vi "ODE_omega.vi"() -> ()   [LabVIEW 2018]
uses:
  <vilib>/imath/engines/lvmath2/RunTimeEngine/BuiltInFunctions/inv/NIMS_inv(GM).vi
  <instcachedir>/0/NIMS_inv(GM)_A6DF8FE880224208AACFE4CF9F659502.lvgen/NIMS_inv(GM)_A6DF8FE880224208AACFE4CF9F659502_000.vi
  <vilib>/imath/engines/lvmath2/RunTimeEngine/ErrorHandling/NIMS_Error From Error Code.vi
  <vilib>/imath/engines/lvmath2/RunTimeEngine/IndexRead/NIMS V(S).vi
  <instcachedir>/0/NIMS V(S)_0488751826AF41519A22953C041130DC.lvgen/NIMS V(S)_0488751826AF41519A22953C041130DC_002.vi
  <vilib>/imathl/engines/lvmath/Functions/Error Handling/Create Error.vi
  <vilib>/imath/engines/lvmath2/RunTimeEngine/ErrorHandling/NIMS_Create Error From Enums.vi
  <vilib>/imath/engines/lvmath2/RunTimeEngine/ArithmeticOperatorToken/NIMS_ArithmeticOperator_multmx-internal.vi
  <instcachedir>/0/NIMS_ArithmeticOperator_multmx-internal_16A6E1DA326644AB974D30232E729C42.lvgen/NIMS_ArithmeticOperator_multmx-internal_16A6E1DA326644AB974D30232E729C42_008.vi
  <vilib>/imath/engines/lvmath2/RunTimeEngine/ArithmeticOperatorToken/NIMS_ArithmeticOperator_multmx(M,CV)-internal.vi
  <instcachedir>/0/NIMS_ArithmeticOperator_multmx(M,CV)-internal_5287250D8D1D4A3E9F77F5DF08D432E0.lvgen/NIMS_ArithmeticOperator_multmx(M,CV)-internal_5287250D8D1D4A3E9F77F5DF08D432E0_003.vi
  <instcachedir>/0/NIMS_ArithmeticOperator_multmx(M,CV)-internal_5287250D8D1D4A3E9F77F5DF08D432E0.lvgen/NIMS_ArithmeticOperator_multmx(M,CV)-internal_5287250D8D1D4A3E9F77F5DF08D432E0_000.vi
  <vilib>/imath/engines/lvmath2/RunTimeEngine/ArithmeticOperatorToken/NIMS_ArithmeticOperator_multmx(M,CV).vi
  <instcachedir>/0/NIMS_ArithmeticOperator_multmx(M,CV)_2F1CD6A2FE4F4213A4AD1C901C2750F5.lvgen/NIMS_ArithmeticOperator_multmx(M,CV)_2F1CD6A2FE4F4213A4AD1C901C2750F5_000.vi
  <vilib>/imath/engines/lvmath2/RunTimeEngine/IndexRead/NIMS M(S).vi
  <instcachedir>/0/NIMS M(S)_B826C018497E4940AE96BD27B540B6FB.lvgen/NIMS M(S)_B826C018497E4940AE96BD27B540B6FB_000.vi
  <vilib>/imath/engines/lvmath2/RunTimeEngine/NodeEndStatement/NIMS_NodeEndStatement_Output.vi
  <instcachedir>/0/NIMS_NodeEndStatement_Output_53EC0D466D134D7ABD903AC30B43404B.lvgen/NIMS_NodeEndStatement_Output_53EC0D466D134D7ABD903AC30B43404B_005.vi
  <vilib>/imath/engines/lvmath2/RunTimeEngine/ErrorHandling/NIMS_Finalize Error.vi
  <vilib>/gmath/NI_Gmath.lvlib
panel:
  out "appended array":dbl[](array[numeric])
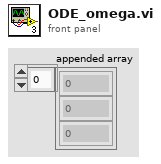
[diagram p1: front panel]
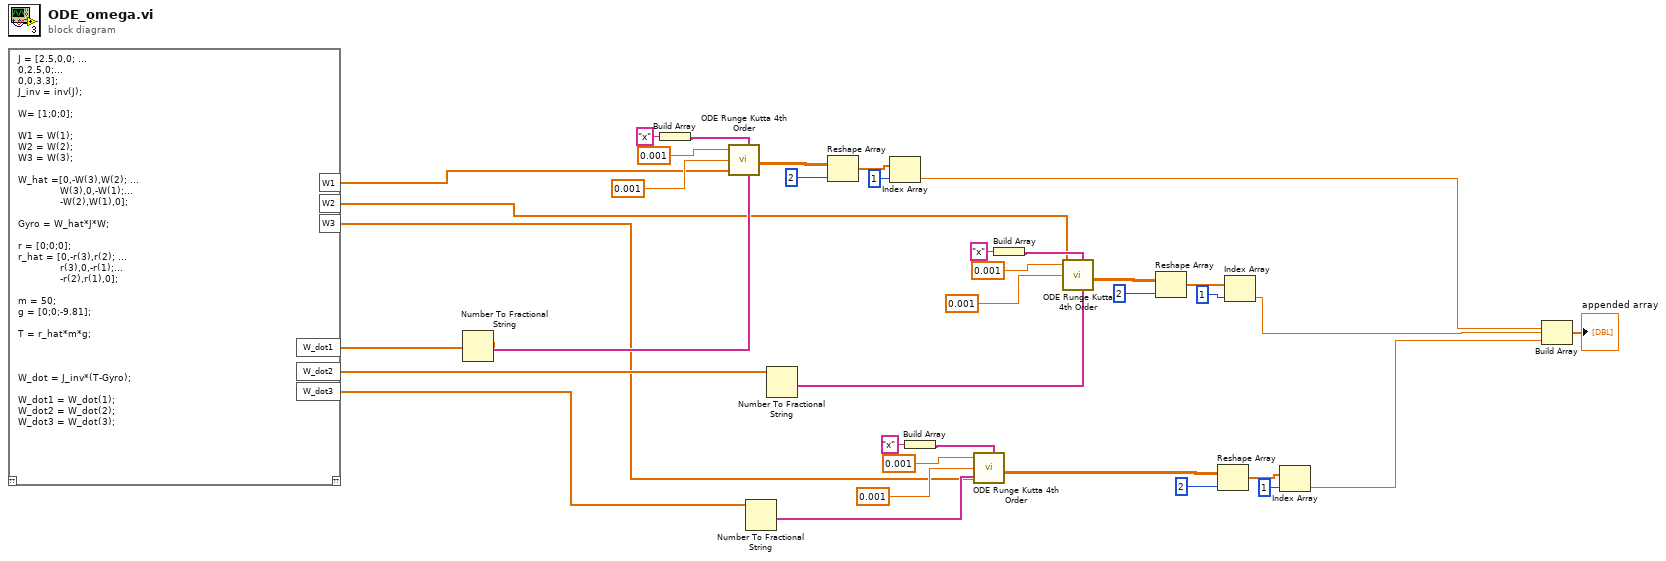
[diagram p0: block diagram]
diagram:
  n1 = mathscript code="J = [2.5,0,0; ...\n0,2.5,0;...\n0,0,3.3];\nJ_inv = inv(J);\n\nW= [1;0;0];\n\nW1 = W(1);\nW2 = W(2);\nW3 = W(3);\n\nW_hat =[0,-W(3),W(2); ...\n              W(3),0,-W(1);...\n              -W(2),W(1),0];\n\nGyro = W_hat*J*W;\n\nr = [0;0;0];\nr_hat = [0,-r(3),r(2); ...\n              r(3),0,-r(1);...\n              -r(2),r(1),0];\n\nm = 50;\ng = [0;0;-9.81];\n\nT = r_hat*m*g;\n\n\n\nW_dot = J_inv*(T-Gyro);\n\nW_dot1 = W_dot(1);\nW_dot2 = W_dot(2);\nW_dot3 = W_dot(3);"() -> ("W_dot1"=w28:dbl[], "W_dot2"=w16:dbl[], "W_dot3"=w5:dbl[], "W1"=w27:dbl[], "W2"=w17:dbl[], "W3"=w6:dbl[])  [unwired: 1 in, 1 out]
  n2 = Number To Fractional String(number=w28) -> (F-format string=w33:string[])  [unwired: 3 in]
  n3 = Build Array("x") -> (w36:string[])
  n4 = call <vilib>:"ODE Runge Kutta 4th Order.vi"("time end"=0.001, "h (step rate)"=0.001, "X0"=w27, "X (name of variables)"=w36, "F(X,t) (right sides of the ODE\nas functions of X and t)"=w33) -> ("X Values (solution)"=w29:dbl[][])  [unwired: 2 in, 3 out]
  n5 = Number To Fractional String(number=w5) -> (F-format string=w11:string[])  [unwired: 3 in]
  n6 = Number To Fractional String(number=w16) -> (F-format string=w22:string[])  [unwired: 3 in]
  n7 = Reshape Array(w29, 2 ("dimension size")) -> (w31:dbl[])
  n8 = Index Array(array=w31, index=1) -> (element=w4:dbl)
  n9 = Build Array("x") -> (w14:string[])
  n10 = call <vilib>:"ODE Runge Kutta 4th Order.vi"("time end"=0.001, "h (step rate)"=0.001, "X0"=w6, "X (name of variables)"=w14, "F(X,t) (right sides of the ODE\nas functions of X and t)"=w11) -> ("X Values (solution)"=w7:dbl[][])  [unwired: 2 in, 3 out]
  n11 = Build Array("x") -> (w25:string[])
  n12 = call <vilib>:"ODE Runge Kutta 4th Order.vi"("time end"=0.001, "h (step rate)"=0.001, "X0"=w17, "X (name of variables)"=w25, "F(X,t) (right sides of the ODE\nas functions of X and t)"=w22) -> ("X Values (solution)"=w18:dbl[][])  [unwired: 2 in, 3 out]
  n13 = Reshape Array(w18, 2 ("dimension size")) -> (w20:dbl[])
  n14 = Reshape Array(w7, 2 ("dimension size")) -> (w9:dbl[])
  n15 = Index Array(array=w20, index=1) -> (element=w3:dbl)
  n16 = Index Array(array=w9, index=1) -> (element=w2:dbl)
  n17 = Build Array(w4, w3, w2) -> (→"appended array":dbl[])
